vi "Combine Channel Output.vi"(8 "error in (no error)":errorcluster, 9 "Enable Channel Combine (T:Enable)":bool=TRUE, 10 "Channel (1:Channel 1)":i32(ring)=1 items=["1"=1, "2"=2], 11 "VISA resource name":refnum<visa-resource-name>) -> (0 "error out":errorcluster, 3 "VISA resource name out":refnum<visa-resource-name>)   [LabVIEW 2015, in "SDG X Series.lvlib"]
doc: "Allows digital data from both channels to added together to create the output signal on the output DAC for the specificd channel."
uses:
  <instrlib>/SDG X Series/SDG X Series.lvlib
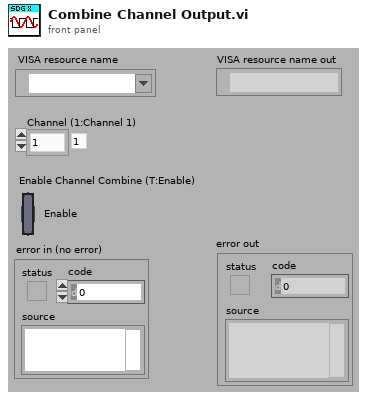
[diagram p1: front panel]
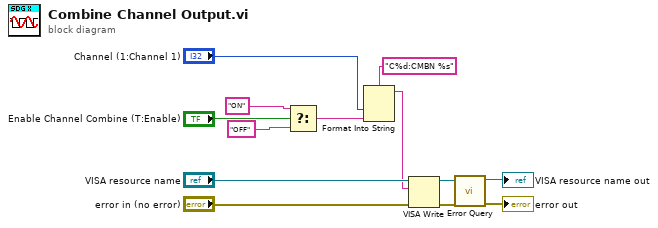
[diagram p0: block diagram]
diagram:
  n1 = Select(t="ON", s="Enable Channel Combine (T:Enable)", f="OFF") -> (s? t:f=w2:string)
  n2 = Format Into String(format string="C%d:CMBN %s", "Channel (1:Channel 1)", w2) -> (resulting string=w5:string)  [unwired: 2 in, 1 out]
  n3 = VISA Write(VISA resource name="VISA resource name", write buffer=w5, error in (no error)="error in (no error)") -> (VISA resource name out=w9:refnum<visa-resource-name>, error out=w7:errorcluster)  [unwired: 1 out]
  n4 = call <instrlib>:"Error Query.vi"("error in (no error)"=w7, "VISA resource name"=w9) -> ("error out"=→"error out":errorcluster, "VISA resource name out"=→"VISA resource name out":refnum<visa-resource-name>)  [unwired: 6 in, 2 out]
